vi "TCPread512B-server.vi"(8 "Error in":errorcluster, 10 "timeout ms (25000)":i32, 11 "connection ID in":refnum<k5>) -> (0 "Error out":errorcluster, 1 "Array":string[](array[string]), 2 "string out":string, 3 "connection ID out":refnum<k5>)   [LabVIEW 2011]
uses:
  <vilib>/regexp/Match Regular Expression.xnode
panel:
  out "match + rest of string":string
  out "Numeric":i32
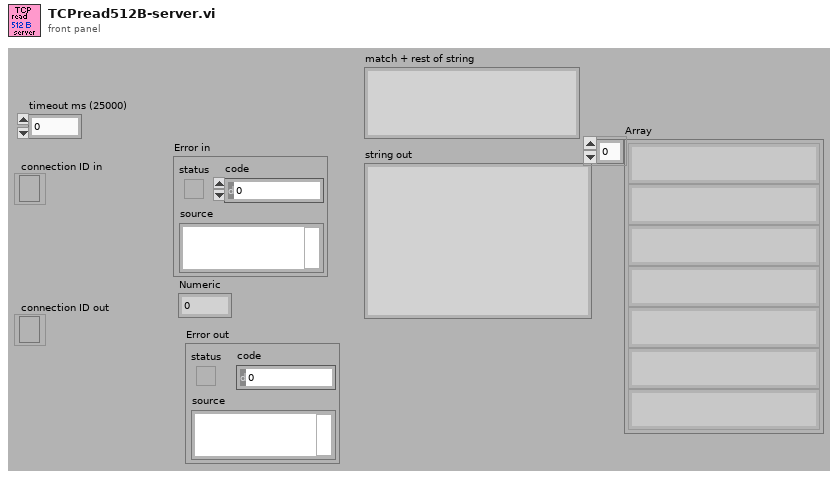
[diagram p1: front panel]
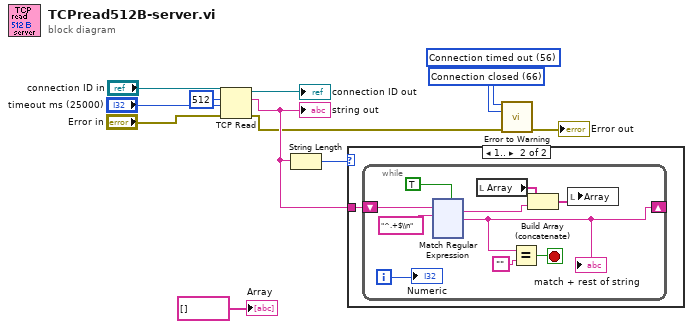
[diagram p0: block diagram]
diagram:
  w1 = 66 items=["No Error", "Argument Error", "Memory Full", "Out of Zone", "End of File", "File Already Open", "Generic File IO Error", "File Not Found", "File Permission Error", "Disk Full", "Duplicate Path", "Too Many Files Open", "Not Enabled", "Resource File Not Found", "Cannot Add Resource", "Resource Not Found", "Image Not Found", "Image Memory Error", "Pen Does Not Exist", "Config Bad Type", "Config Token Not Found", "Config Parse Error", "Config Memory Error", "Bad External Code Format", "Bad External Code Offset", "External Code Not Present", "Null Window", "Destroy Window Mixup", "Null Menu", "Print Aborted", "Bad Print Record", "Print Driver Error", "Windows Error During Print", "Memory Error During Print", "Print Dialog Error", "Generic Print Error", "Invalid Device Refnum", "Device Not Found", "Device Parameter Error", "Device Unit Error", "Can't Open Device", "Device Call Aborted", "Generic Error", "Cancelled By User", "Object ID Too Low", "Object ID Too High", "Object Not In Heap", "Unknown Heap", "Bad DefProc ID", "DefProc Not In Table", "Message Out Of Range", "Null Method", "Unknown Message", "Manager Call Not Supported", "Bad address", "Connection In progress", "Connection timed out", "Connection is already in progress", "Network attribute not supported", "Network error", "Address in use", "System out of memory", "Connection aborted", "Connection refused", "Connection is not connected", "Connection is already connected", "Connection closed", "Initialize error (interapplication manager)", "Bad occurrence", "Wait on unbound occurrence handler", "Occurrence queue overflow", "Bad path", "Semaphore not signaled", "Unrecognized type (interapplication manager)"] ("2nd Error to Convert")
  w3 = 56 items=["No Error", "Argument Error", "Memory Full", "Out of Zone", "End of File", "File Already Open", "Generic File IO Error", "File Not Found", "File Permission Error", "Disk Full", "Duplicate Path", "Too Many Files Open", "Not Enabled", "Resource File Not Found", "Cannot Add Resource", "Resource Not Found", "Image Not Found", "Image Memory Error", "Pen Does Not Exist", "Config Bad Type", "Config Token Not Found", "Config Parse Error", "Config Memory Error", "Bad External Code Format", "Bad External Code Offset", "External Code Not Present", "Null Window", "Destroy Window Mixup", "Null Menu", "Print Aborted", "Bad Print Record", "Print Driver Error", "Windows Error During Print", "Memory Error During Print", "Print Dialog Error", "Generic Print Error", "Invalid Device Refnum", "Device Not Found", "Device Parameter Error", "Device Unit Error", "Can't Open Device", "Device Call Aborted", "Generic Error", "Cancelled By User", "Object ID Too Low", "Object ID Too High", "Object Not In Heap", "Unknown Heap", "Bad DefProc ID", "DefProc Not In Table", "Message Out Of Range", "Null Method", "Unknown Message", "Manager Call Not Supported", "Bad address", "Connection In progress", "Connection timed out", "Connection is already in progress", "Network attribute not supported", "Network error", "Address in use", "System out of memory", "Connection aborted", "Connection refused", "Connection is not connected", "Connection is already connected", "Connection closed", "Initialize error (interapplication manager)", "Bad occurrence", "Wait on unbound occurrence handler", "Occurrence queue overflow", "Bad path", "Semaphore not signaled", "Unrecognized type (interapplication manager)"] ("1st Error to Convert")
  n1 = TCP Read ("TCP Read Command")(connection ID="connection ID in", bytes to read=512, error in (no error)="Error in", 9:"timeout ms (25000)") -> (connection ID out=→"connection ID out":refnum<k5>, data out=w6:string, error out=w5:errorcluster)  [unwired: 1 out]
  "string out" <- w6
  n2 = String Length(string=w6) -> (length=w7:i32)
  n3 = case shown="1.." w7 {
    tunnel: w6 -> [_ w13]
    frame ..0 {
    }
    frame 1.. {
      n4 = while {
        shift-right: [w15] -> _
        shift-left: w13 -> [w14]
        i -> [w23]
        stop <- w19 stop-if-true
        n5 = xnode "Match Regular Expression"("input string"=w14, "regular expression"="^.+$\\n", "multiline? (F)"=TRUE) -> ("whole match"=w16:string, "after match"=w15:string)  [unwired: 2 in, 4 out]
        "match + rest of string" <- w15
        n6 = local read "Array"() -> (w21:string[])
        n7 = Equal?(x=w15, y="") -> (x = y?=w19:bool)
        n8 = Build Array (concatenate)(w21, w16) -> (w22:string[])
        n9 = local write "Array"(w22) -> ()
        "Numeric" <- w23
      }
    }
  }
  n10 = call <vilib>:"Error to Warning.vi"("1st Error to Convert"=w3, "2nd Error to Convert"=w1, "error in"=w5) -> ("warning out"=→"Error out":errorcluster)  [unwired: 2 in, 10 out]
  "Array" <- string[] []
